vi "Setup_Pictures_Plots.vi"(3 "Picture Dim":i16[](array[numeric]), 4 "Plot Axis":T1, 5 "Picture In":picture) -> (1 "Draw Area Size":cluster{u32, u32}, 2 "Picture Out":picture)   [LabVIEW 2010]
uses:
  Pict_Plot_Axis.ctl
  Axis.ctl
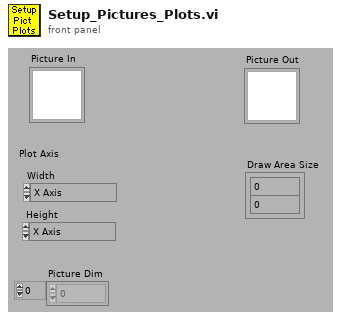
[diagram p1: front panel]
types:
  T1 = typedef "Pict_Plot_Axis.ctl" = cluster{"Width":T2, "Height":T2}
  T2 = typedef "Axis.ctl" = enum16{"X Axis", "X Axis -ve", "Y Axis", "Y Axis -ve", "Z Axis", "Z Axis -ve"}
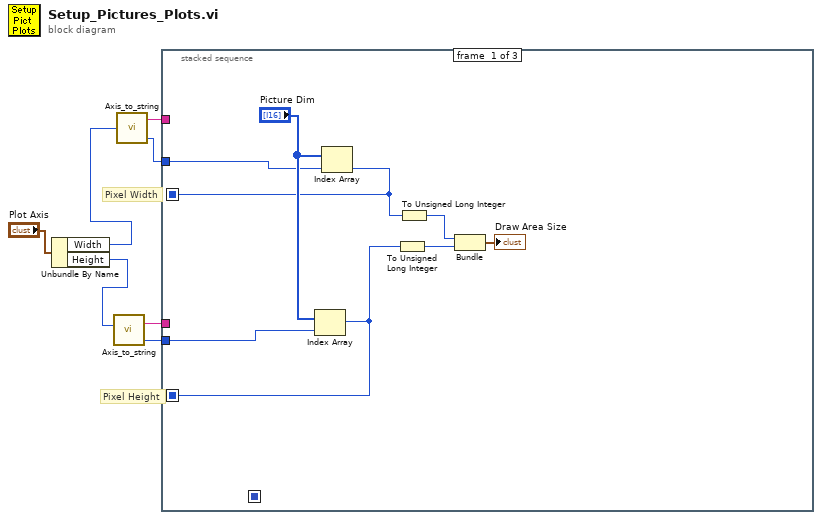
[diagram p0: block diagram]
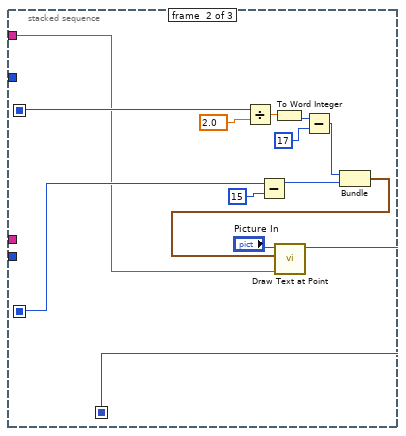
[diagram p2: hidden frame]
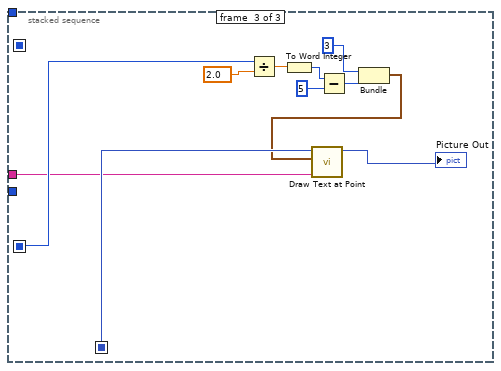
[diagram p3: hidden frame]
diagram:
  # "Pixel Height"
  # "Pixel Width"
  n1 = Unbundle By Name("Plot Axis") -> ("Width"=w2:T2, "Height"=w1:T2)
  n2 = call "Axis_to_string.vi"("Axis"=w1) -> ("String"=w4:string, "Index"=w6:i32)  [unwired: 1 out]
  n3 = call "Axis_to_string.vi"("Axis"=w2) -> ("String"=w5:string, "Index"=w7:i32)  [unwired: 1 out]
  n4 = stacked-sequence {
    seq-local: [w13 _ _] -> [_ w19 _]
    seq-local: [w14 _ _] -> [_ w17 w31]
    seq-local: [_ w18 _] -> [_ _ w33]
    tunnel: w7 -> [w11 _ _]
    tunnel: w6 -> [w10 _ _]
    tunnel: w5 -> [_ w16 _]
    tunnel: w4 -> [_ _ w30]
    frame #0 {
      n5 = Index Array(array="Picture Dim", index=w10) -> (element=w14:i16)
      n6 = Index Array(array="Picture Dim", index=w11) -> (element=w13:i16)
      n7 = To Unsigned Long Integer(number=w14) -> (unsigned 32bit integer=w9:u32)
      n8 = To Unsigned Long Integer(number=w13) -> (unsigned 32bit integer=w8:u32)
      n9 = Bundle(w8, w9) -> (→"Draw Area Size":cluster{u32, u32})  [unwired: 1 out]
    }
    frame #1 {
      n10 = Divide(x=w19, y=2.0) -> (x/y=w22:dbl)
      n11 = Subtract(x=w17, y=i16 15) -> (x-y=w24:i16)
      n12 = To Word Integer(number=w22) -> (16bit integer=w26:i16)
      n13 = Subtract(x=w26, y=i16 17) -> (x-y=w28:i16)
      n14 = Bundle(w28, w24) -> (w25:cluster{i16, i16})  [unwired: 1 out]
      n15 = call <vilib>:"Draw Text at Point.vi"("text"=w16, "origin"=w25, "picture"="Picture In") -> ("new picture"=w18:picture)  [unwired: 6 in, 2 out]
    }
    frame #2 {
      n16 = Divide(x=w31, y=2.0) -> (x/y=w35:dbl)
      n17 = To Word Integer(number=w35) -> (16bit integer=w37:i16)
      n18 = Subtract(x=w37, y=i16 5) -> (x-y=w38:i16)
      n19 = Bundle("32bit integer"=i16 3, w38) -> (w32:cluster{"32bit integer":i16, i16})  [unwired: 1 out]
      n20 = call <vilib>:"Draw Text at Point.vi"("text"=w30, "origin"=w32, "picture"=w33) -> ("new picture"=→"Picture Out":picture)  [unwired: 6 in, 2 out]
    }
  }
